vi "Data_get_joe_2.vi"() -> ()   [LabVIEW 2011]
uses:
  <vilib>/Utility/error.llb/DialogType.ctl
  <vilib>/Analysis/2dsp.llb/Real FFT.vi
  <vilib>/Analysis/NI_AALPro.lvlib
panel:
  in  "Automatic Overwrite?":bool
  out "f cur. (GHz)":i32
  in  "TDS VISA Port":refnum<visa-resource-name>="GPIB0::1::INSTR"
  in  "Chirp up to (GHz)":dbl
  in  "PauseB":bool caption="Pause"
  in  "Substr":bool
  out "tdsavges#":i32 caption="tds averaged:"
  in  "Auto":bool caption="Autosave"
  in  "FFT every#":u32=1 min=1 max=1000 step=1
  in  "#steps":u32=1 min=1 step=1
  in  "f step (MHz)":dbl=0.0003 min=0.00025 max=67.0 step=1e-06 format="%#.12f"
  in  "time/point":T1(ring)
  in  "time/div":T2(ring)
  out "Current sweep":u32=1 min=1 max=1000 step=1
  in  "Ext":string="ccd"
  in  "Name":string="trace"
  in  "Folder":path
  in  "#Sweeps":u32=1 min=1 max=1000 step=1
  in  "Ampl. (dBm)":dbl min=-135.0 max=30.0 step=0.5 format="%#_8g"
  in  "f start (GHz)":dbl=0.0003 min=0.00025 max=67.0 step=1e-06 format="%#.12f"
  in  "Start":bool
  in  "Quit":bool
  in  "Visa Port":refnum<visa-resource-name>="GPIB0::1::INSTR"
  out "read time (ms)":u32
  out "#points":u32
  out "Busy":bool
  in  "Chirp start (MHz)":ext=2.5
  in  "Filter up to (MHz)":ext=2.5
  in  "Amount of averagings":u32=10 min=1 step=1
  out "Data":dbl[](array[numeric])
  out "Frequency Domain Signal":cluster{ext[], dbl[]}(graph)
  out "FFT (Im)":dbl[](array[numeric])
  out "FFT (Re)":dbl[](array[numeric])
  out "Final array":ext[][](array[numeric])
  out "size(s)":i32
  out "Oscilloscope Data":dbl[](array[numeric])
  in  "Channel Number":u16=1
  out "Oscilloscope graph":dbl[](graph)
  in  "Stop":bool
  # "Oscilloscope TDS6124C"
  # "File Storage"
  # "PSG E8257D"
  # "Control"
  # "Spectrum data"
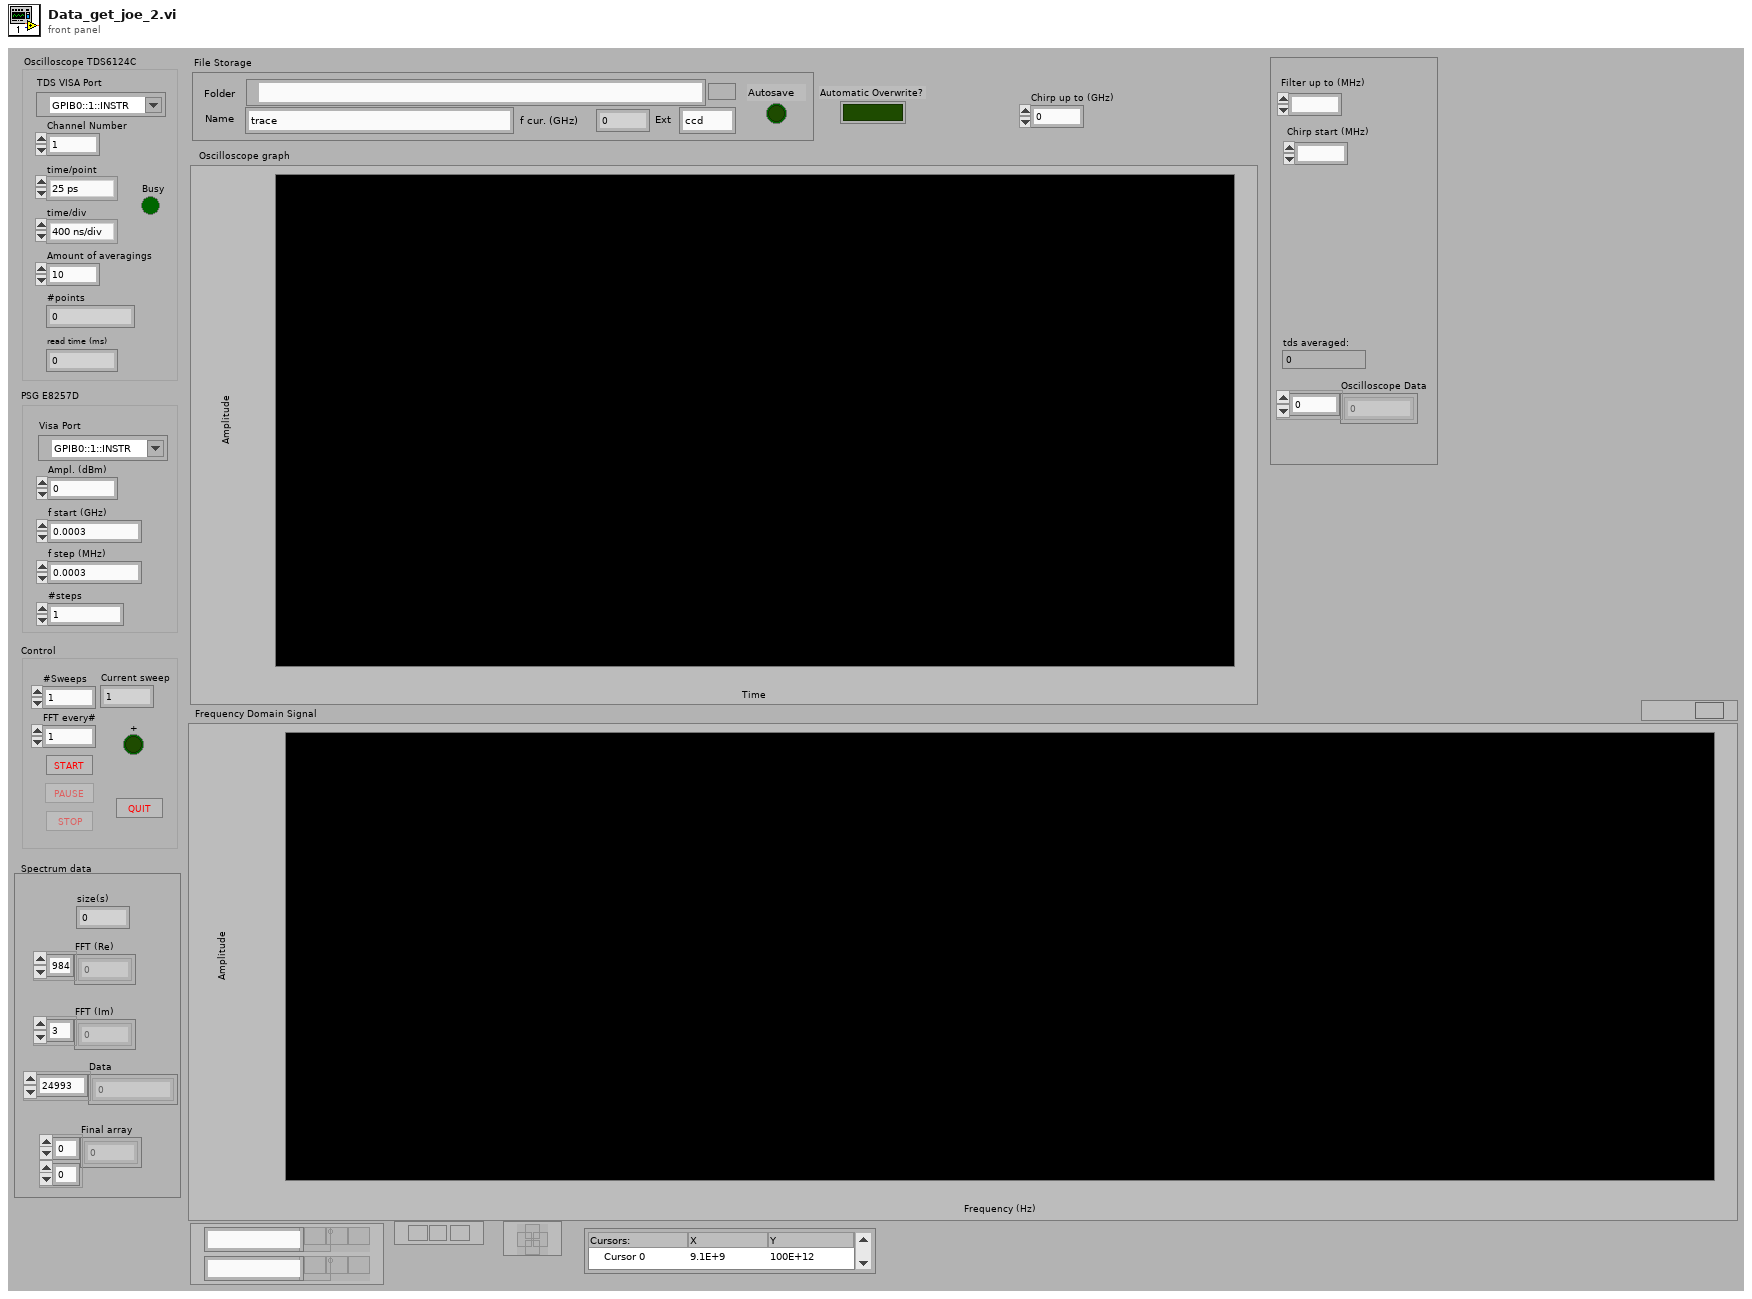
[diagram p1: front panel]
types:
  T1 = enum16{"25 ps", "50 ps", "100 ps", "200 ps", "400 ps", "800 ps", "2 ns"}
  T2 = enum16{"400 ns/div", "1 us/div", "2 us/div", "4 us/div", "10 us/div", "20 us/div"}
  T3 = enum8{"Enabled", "Disabled", "Disabled and Grayed Out"}
  T4 = enum16{"open", "replace", "create", "open or create", "replace or create", "replace or create with confirmation"}
  T5 = typedef "DialogType.ctl" = u16
  T6 = cluster{"Folder":path, "Name":string, "Ext":string}
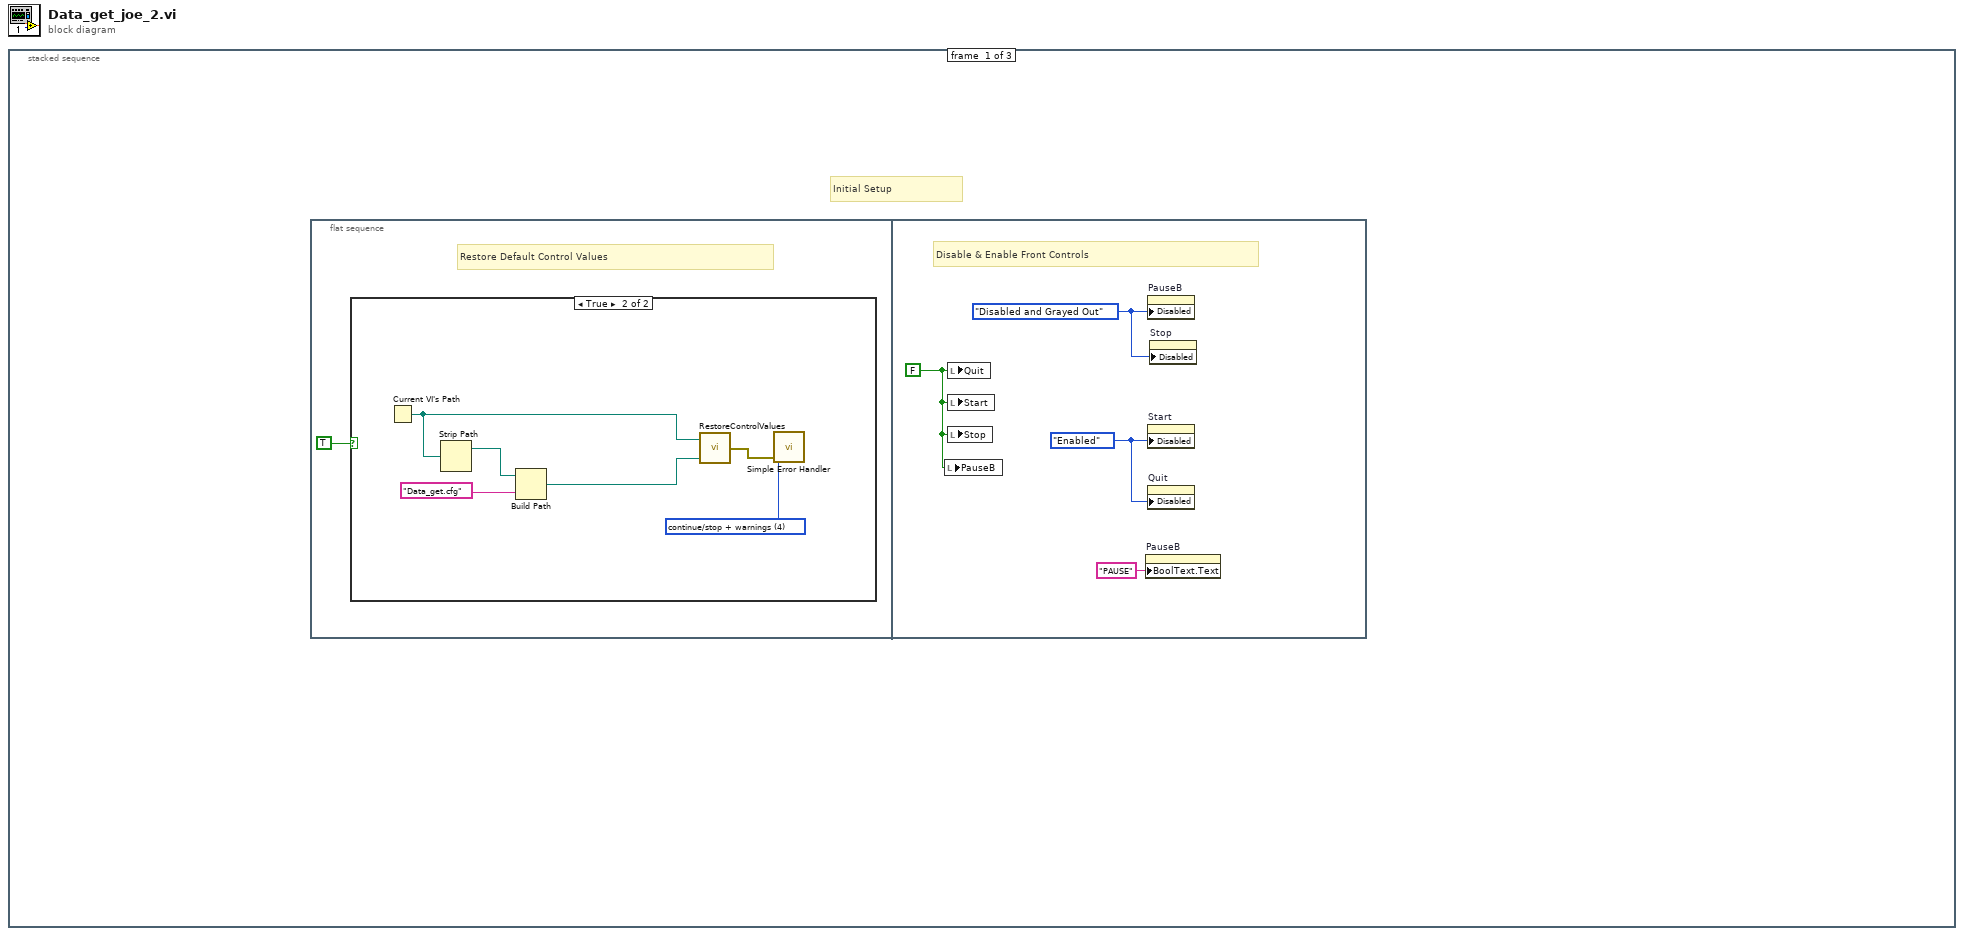
[diagram p0: block diagram]
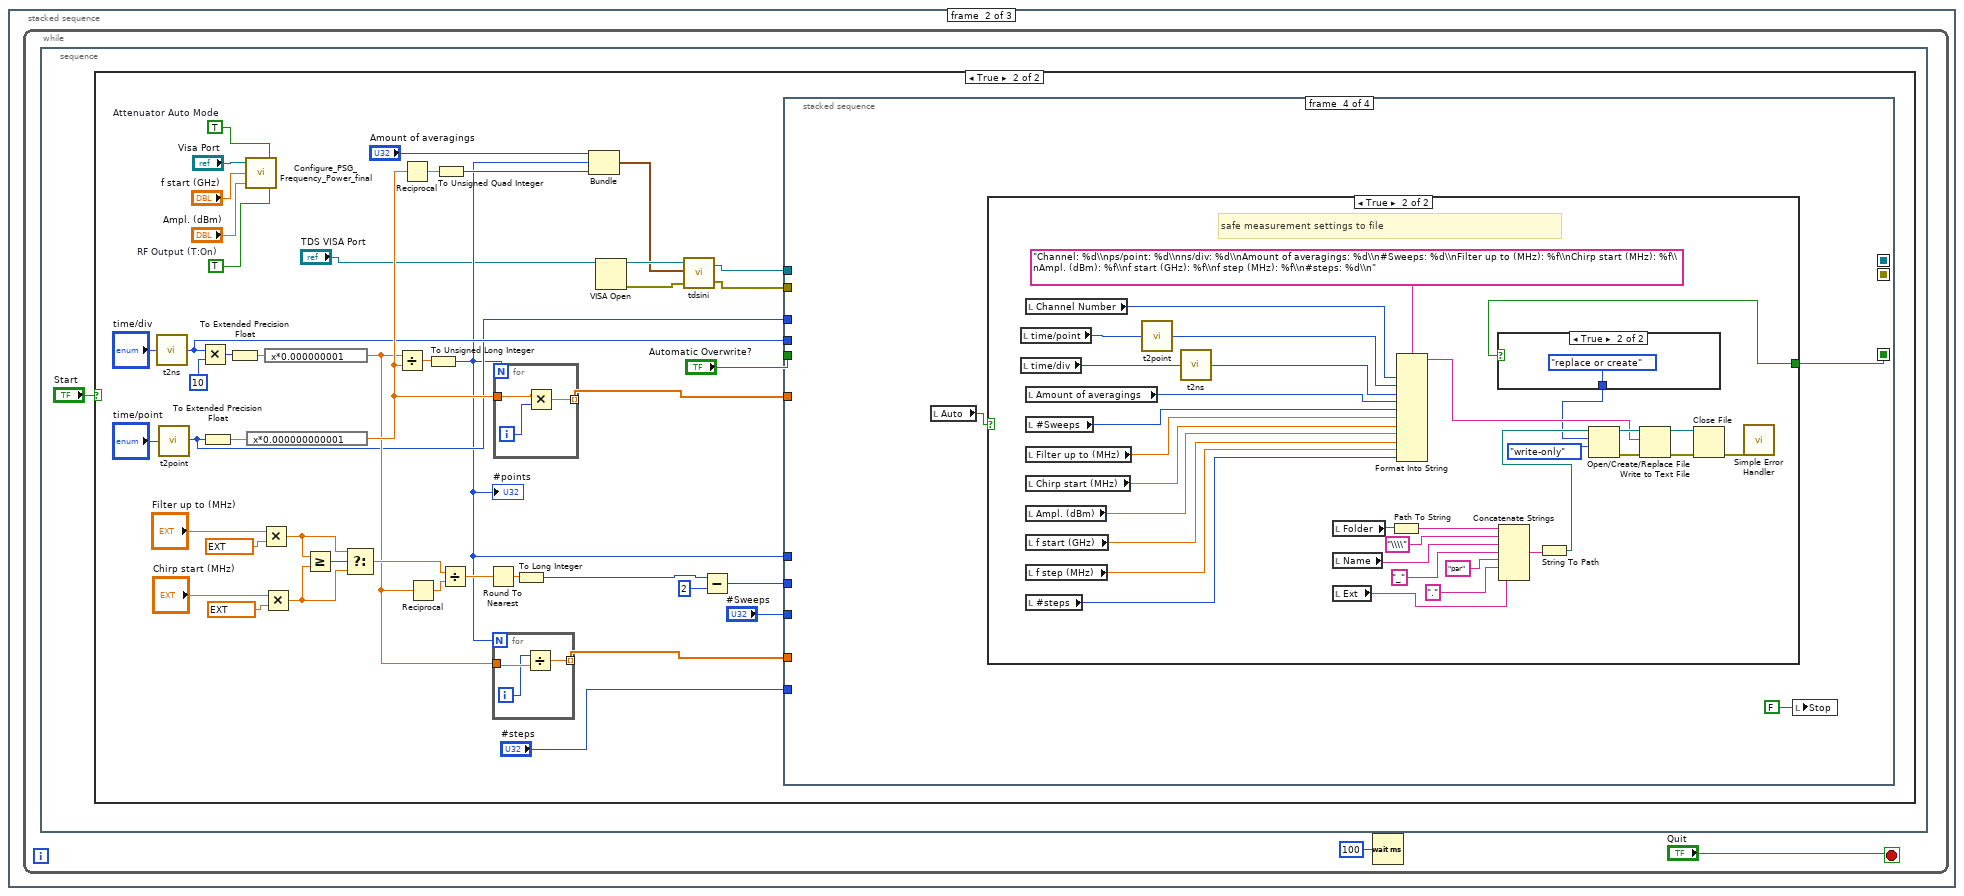
[diagram p3: hidden frame]
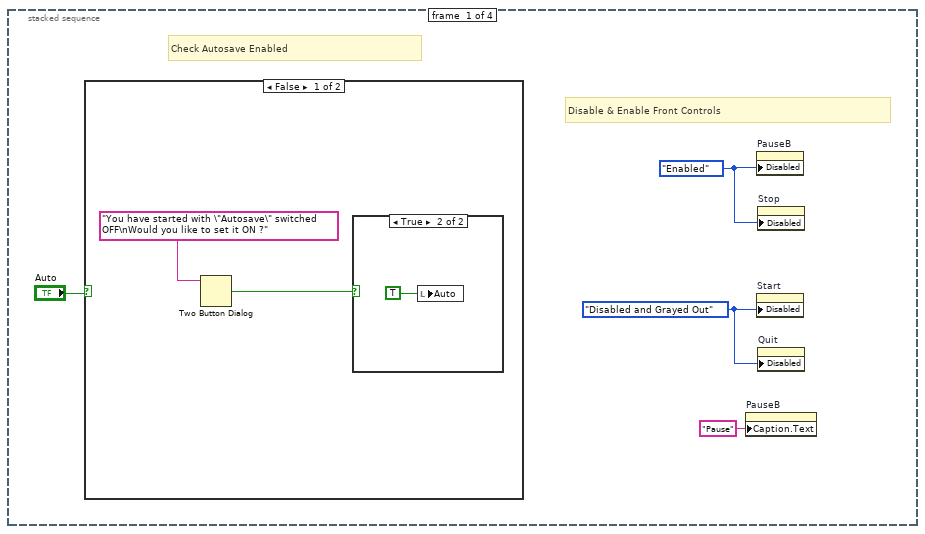
[diagram p5: hidden frame]
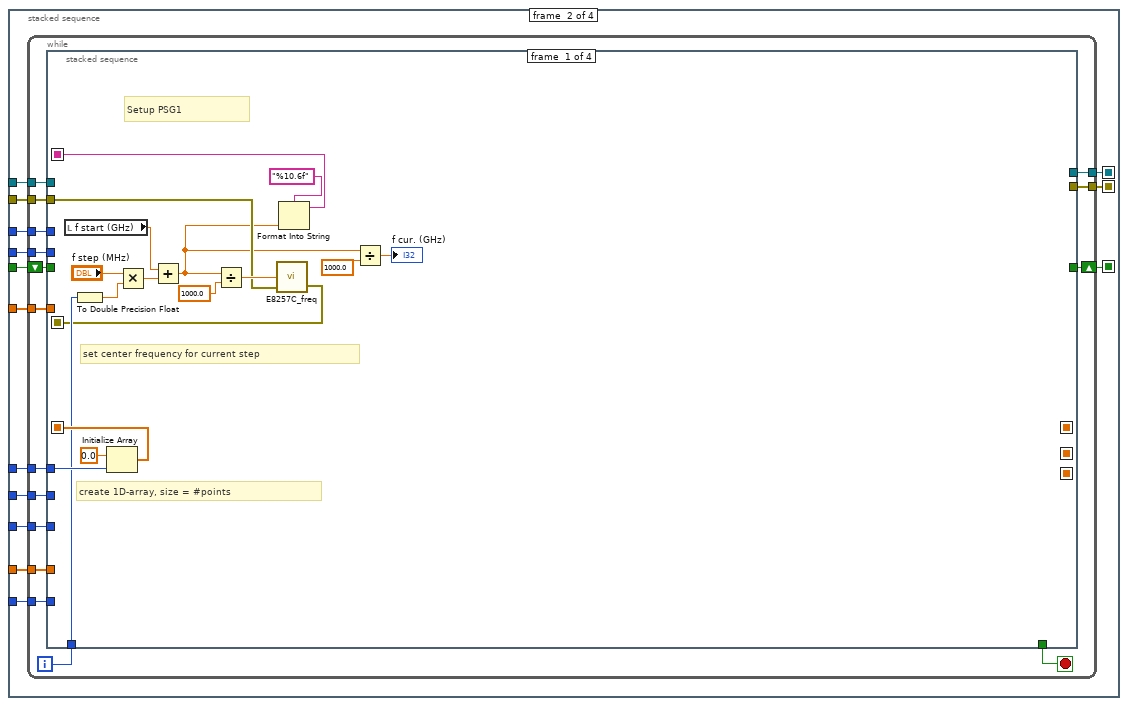
[diagram p8: hidden frame]
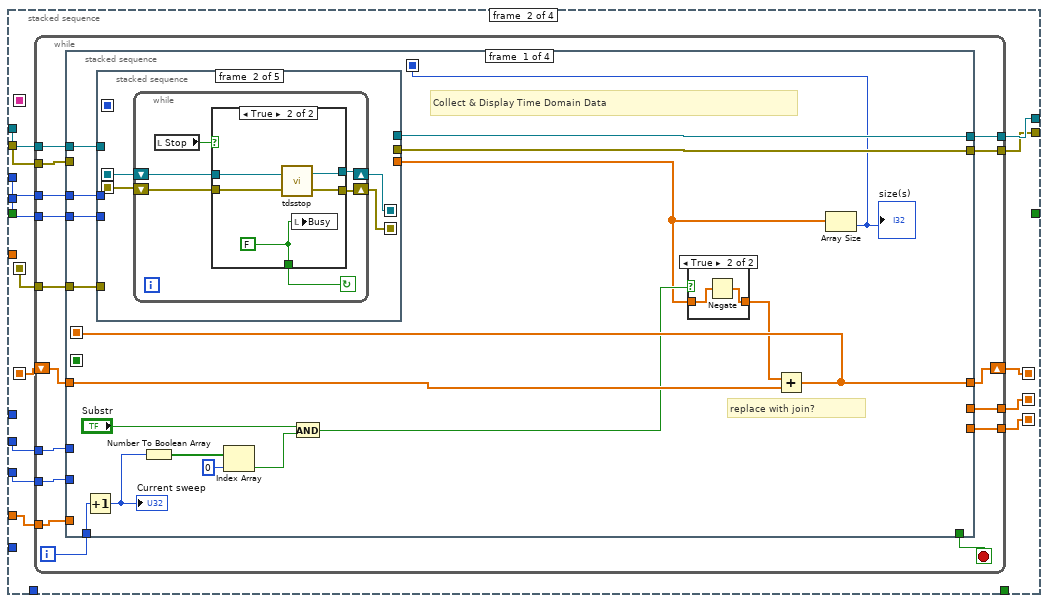
[diagram p9: hidden frame]
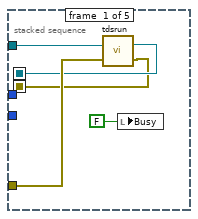
[diagram p11: hidden frame]
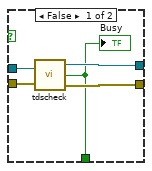
[diagram p12: hidden frame]
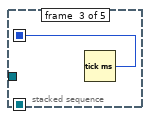
[diagram p13: hidden frame]
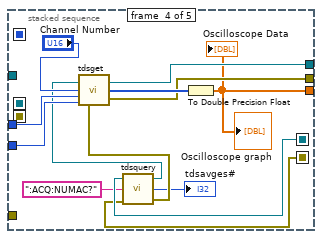
[diagram p14: hidden frame]
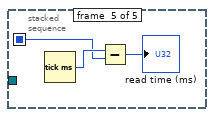
[diagram p15: hidden frame]
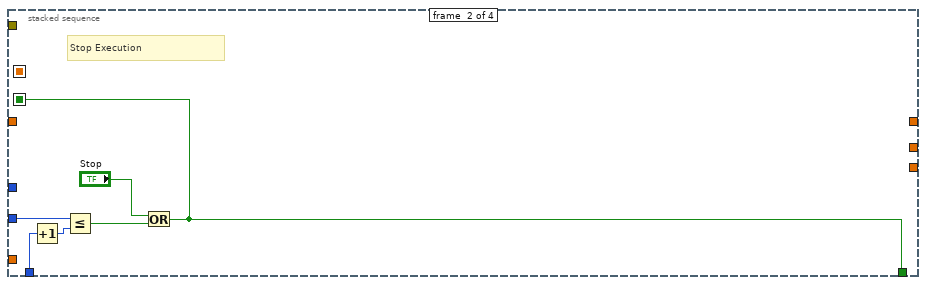
[diagram p16: hidden frame]
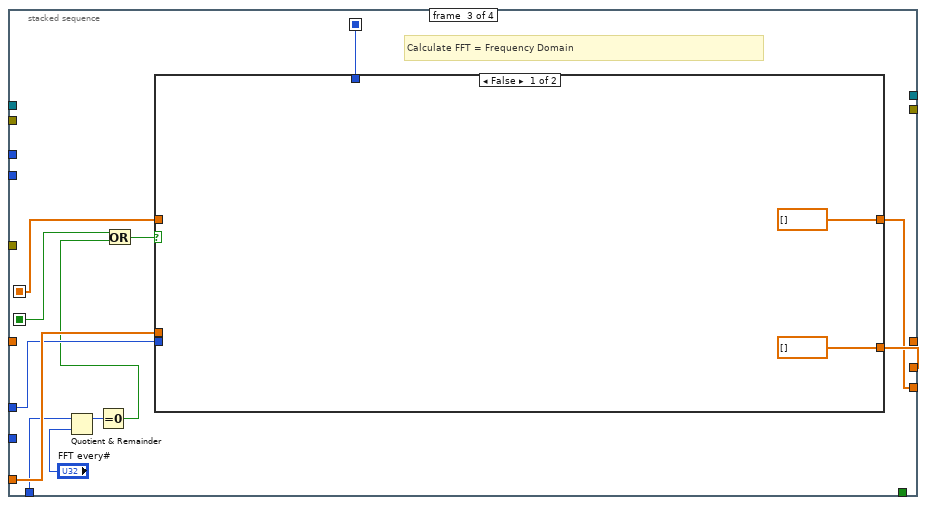
[diagram p17: hidden frame]
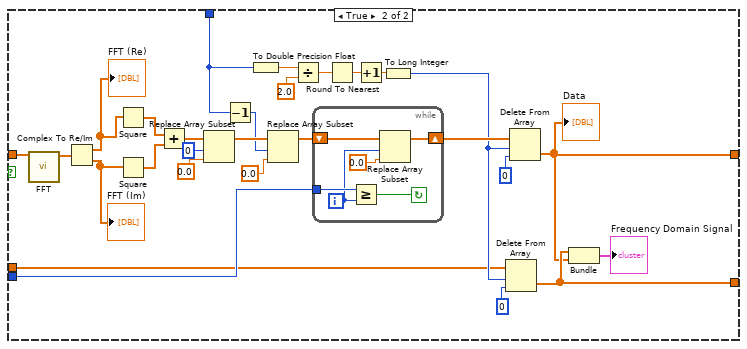
[diagram p18: hidden frame]
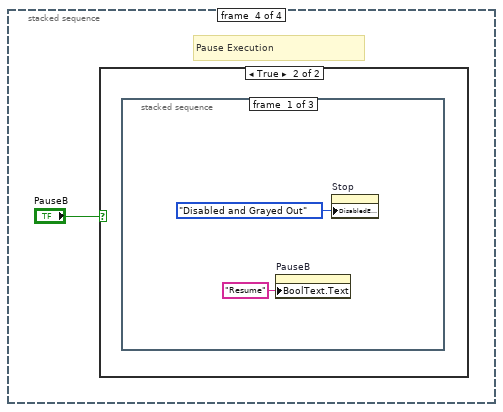
[diagram p19: hidden frame]
diagram:
  n1 = stacked-sequence {
    frame #0 {
      # "Initial Setup"
      n2 = flat-sequence {
        frame #0 {
          # "Restore Default Control Values"
          n3 = case shown="True" TRUE {
            frame False {
            }
            frame True {
              w2 = T5 4 items=["no dialog", "OK message", "continue or stop message", "OK message + warnings", "continue/stop + warnings"] ("type of dialog (OK msg:1)")
              n4 = Current VI's Path() -> (path=w3:path)
              n5 = Strip Path(path=w3) -> (stripped path=w4:path)  [unwired: 1 out]
              n6 = Build Path(base path=w4, name or relative path="Data_get.cfg") -> (appended path=w6:path)
              n7 = call "RestoreControlValues.vi"("file path"=w6, "vi path"=w3) -> ("error out"=w5:errorcluster)
              n8 = call <vilib>:"Simple Error Handler.vi"("type of dialog (OK msg:1)"=w2, "error in (no error)"=w5) -> ()  [unwired: 3 in, 5 out]
            }
          }
        }
        frame #1 {
          w10 = T3."Disabled and Grayed Out" ("Disabled")
          w8 = T3."Enabled" ("Disabled")
          w11 = FALSE ("Quit")
          # "Disable & Enable Front Controls"
          n9 = local write "PauseB"(w11) -> ()
          n10 = local write "Quit"(w11) -> ()
          n11 = local write "Start"(w11) -> ()
          n12 = local write "Stop"(w11) -> ()
          n13 = property on="PauseB" class="Bool (strict)"("BoolText.Text"="PAUSE" ("Boolean Text.Text")) -> ()  [unwired: 2 in, 2 out]
          n14 = property on="PauseB" class="Bool (strict)"("Disabled"=w10) -> ()  [unwired: 2 in, 2 out]
          n15 = property on="Start" class="Bool (strict)"("Disabled"=w8) -> ()  [unwired: 2 in, 2 out]
          n16 = property on="Quit" class="Bool (strict)"("Disabled"=w8) -> ()  [unwired: 2 in, 2 out]
          n17 = property on="Stop" class="Bool (strict)"("Disabled"=w10) -> ()  [unwired: 2 in, 2 out]
        }
      }
    }
    frame #1 {
      n18 = while {
        stop <- "Quit" stop-if-true
        n19 = stacked-sequence {
          frame #0 {
            n20 = case shown="True" "Start" {
              frame False {
              }
              frame True {
                w19 = TRUE  # Attenuator Auto Mode
                w16 = TRUE  # RF Output (T:On)
                n21 = call "t2ns.vi"("t/div"="time/div") -> ("ns/div"=w31:u32)
                n22 = call "t2point.vi"("t/point"="time/point") -> ("ps/point"=w29:u32)
                n23 = Multiply(x=w31, y=u32 10) -> (x*y=w54:u32)
                n24 = To Extended Precision Float(1:w29) -> (0:w51:ext)
                n25 = To Extended Precision Float(1:w54) -> (0:w52:ext)
                n26 = call "Configure_PSG_ Frequency_Power_final.vi"("RF Output (T:On)"=w16, "Attenuator Auto Mode (T:Enable)"=w19, "Power [dBm]"="Ampl. (dBm)", "Frequency [GHz]"="f start (GHz)", "VISA resource name"="Visa Port") -> ()
                n27 = expression code="x*0.000000000001"(w51) -> (w37:ext)
                n28 = Multiply(x="Filter up to (MHz)", y=ext 1000000.0) -> (x*y=w43:ext)
                n29 = Multiply(x="Chirp start (MHz)", y=ext 1000000.0) -> (x*y=w40:ext)
                n30 = expression code="x*0.000000001"(w52) -> (w33:ext)
                n31 = Greater Or Equal?(x=w43, y=w40) -> (x >= y?=w50:bool)
                n32 = Select(t=w43, s=w50, f=w40) -> (s? t:f=w48:ext)
                n33 = Divide(x=w33, y=w37) -> (x/y=w53:ext)
                n34 = Reciprocal(x=w37) -> (1/x=w35:ext)
                n35 = Reciprocal(x=w33) -> (1/x=w49:ext)
                n36 = To Unsigned Long Integer(number=w53) -> (unsigned 32bit integer=w27:u32)
                "#points" <- w27
                n37 = To Unsigned Quad Integer(1:w35) -> (0:w36:u64)
                n38 = Divide(x=w48, y=w49) -> (x/y=w47:ext)
                n39 = Round To Nearest(number=w47) -> (nearest integer value=w46:ext)
                n40 = for {
                  N: w27 -> [_]
                  tunnel: w33 -> [w459]
                  tunnel: [w460] -> w34 mode=indexing
                  i -> [w458]
                  n41 = Divide(x=w458, y=w459) -> (x/y=w460:ext)
                }
                n42 = for {
                  N: w27 -> [_]
                  tunnel: w37 -> [w463]
                  tunnel: [w462] -> w32 mode=indexing
                  i -> [w461]
                  n43 = Multiply(x=w463, y=w461) -> (x*y=w462:ext)
                }
                n44 = To Long Integer(number=w46) -> (32bit integer=w24:i32)
                n45 = Bundle("Amount of averagings"="Amount of averagings", w27, w36) -> (w38:cluster{"Amount of averagings ":u32, u32, u64})  [unwired: 1 in]
                n46 = VISA Open(VISA resource name="TDS VISA Port") -> (VISA resource name=w56:refnum<visa-resource-name>, error out=w57:errorcluster)  [unwired: 4 in]
                n47 = call "tdsini.vi"("Error In (No Error)"=w57, "Acq_par"=w38, "VISA Port In"=w56) -> ("Error Out"=w58:errorcluster, "VISA Port Out"=w59:refnum<visa-resource-name>)
                n48 = Subtract(x=w24, y=2) -> (x-y=w22:i32)
                n49 = stacked-sequence {
                  seq-local: [_ w73 _ _] -> [_ _ w419 _]
                  seq-local: [_ w72 _ _] -> [_ _ w418 _]
                  seq-local: [_ w67 _ _] -> [_ _ _ w420]
                  tunnel: w59 -> [_ w80 _ _]
                  tunnel: w58 -> [_ w79 _ _]
                  tunnel: w29 -> [_ w78 _ _]
                  tunnel: w31 -> [_ w77 _ _]
                  tunnel: w22 -> [_ w76 _ _]
                  tunnel: w34 -> [_ w75 _ _]
                  tunnel: "#Sweeps" -> [_ w74 _ _]
                  tunnel: w32 -> [_ w69 _ _]
                  tunnel: w27 -> [_ w71 _ _]
                  tunnel: "#steps" -> [_ w70 _ _]
                  tunnel: "Automatic Overwrite?" -> [_ w68 _ _]
                  frame #0 {
                    w61 = T3."Enabled" ("Disabled")
                    w60 = T3."Disabled and Grayed Out" ("Disabled")
                    # "Check Autosave Enabled"
                    # "Disable & Enable Front Controls"
                    n50 = case shown="False" "Auto" {
                      frame False {
                        n51 = Two Button Dialog(message="You have started with \"Autosave\" switched OFF\nWould you like to set it ON ?") -> (T button?=w64:bool)  [unwired: 2 in]
                        n52 = case shown="True" w64 {
                          frame False {
                          }
                          frame True {
                            n53 = local write "Auto"(TRUE) -> ()
                          }
                        }
                      }
                      frame True {
                      }
                    }
                    n54 = property on="PauseB" class="Bool (strict)"("Caption.Text"="Pause") -> ()  [unwired: 2 in, 2 out]
                    n55 = property on="PauseB" class="Bool (strict)"("Disabled"=w61) -> ()  [unwired: 2 in, 2 out]
                    n56 = property on="Start" class="Bool (strict)"("Disabled"=w60) -> ()  [unwired: 2 in, 2 out]
                    n57 = property on="Stop" class="Bool (strict)"("Disabled"=w61) -> ()  [unwired: 2 in, 2 out]
                    n58 = property on="Quit" class="Bool (strict)"("Disabled"=w60) -> ()  [unwired: 2 in, 2 out]
                  }
                  frame #1 {
                    n59 = while {
                      tunnel: w80 -> [w96]
                      tunnel: w79 -> [w95]
                      tunnel: w78 -> [w94]
                      tunnel: w77 -> [w93]
                      tunnel: w76 -> [w92]
                      tunnel: w75 -> [w91]
                      tunnel: w74 -> [w90]
                      tunnel: [w89] -> w73
                      tunnel: [w88] -> w72
                      tunnel: w71 -> [w87]
                      tunnel: w70 -> [w85]
                      tunnel: w69 -> [w83]
                      shift-right: [w81] -> w67
                      shift-left: w68 -> [w82]
                      i -> [w86]
                      stop <- w84 stop-if-true
                      n60 = stacked-sequence {
                        seq-local: [w112 _ _ _] -> [_ w118 _ _]
                        seq-local: [w102 _ _ _] -> [_ w117 _ _]
                        seq-local: [_ w116 _ _] -> [_ _ w274 _]
                        seq-local: [_ w115 _ _] -> [_ _ w273 _]
                        seq-local: [_ w114 _ _] -> [_ _ w272 _]
                        seq-local: [w100 _ _ _] -> [_ _ w271 _]
                        tunnel: w96 -> [_ w127 _ _]
                        tunnel: w95 -> [w103 w126 _ _]
                        tunnel: w94 -> [_ w125 _ _]
                        tunnel: w93 -> [_ w124 _ _]
                        tunnel: w92 -> [_ w123 _ _]
                        tunnel: w91 -> [_ w122 _ _]
                        tunnel: w90 -> [_ w121 _ _]
                        tunnel: [_ w120 _ _] -> w89
                        tunnel: [_ w119 _ _] -> w88
                        tunnel: w87 -> [w111 _ _ _]
                        tunnel: w86 -> [w106 _ _ w412]
                        tunnel: w85 -> [_ _ _ w411]
                        tunnel: [_ _ _ w410] -> w84
                        tunnel: w83 -> [_ _ w275 _]
                        tunnel: w82 -> [_ _ w269 _]
                        tunnel: [_ _ w268 _] -> w81
                        frame #0 {
                          # "Setup PSG1"
                          # "create 1D-array, size = #points"
                          # "set center frequency for current step"
                          n61 = local read "f start (GHz)"() -> (w104:dbl)
                          n62 = To Double Precision Float(number=w106) -> (double precision float=w107:dbl)
                          n63 = Initialize Array(0.0 ("element"), w111) -> (w112:dbl[])
                          n64 = Multiply(x="f step (MHz)", y=w107) -> (x*y=w105:dbl)
                          n65 = Add(x=w104, y=w105) -> (x+y=w98:dbl)
                          n66 = Divide(x=w98, y=1000.0) -> (x/y=w110:dbl)
                          n67 = call "E8257C_freq.vi"("error in"=w103, "Frequency GHz"=w110) -> ("error out"=w102:errorcluster)  [unwired: 1 in]
                          n68 = Format Into String(format string="%10.6f", w98) -> (resulting string=w100:string)  [unwired: 2 in, 1 out]
                          n69 = Divide(x=w98, y=1000.0) -> (x/y=→"f cur. (GHz)":dbl)
                        }
                        frame #1 {
                          n70 = while {
                            tunnel: [w140] -> w119
                            tunnel: [w141] -> w120
                            tunnel: w126 -> [w142]
                            tunnel: w127 -> [w143]
                            tunnel: w125 -> [w139]
                            tunnel: w124 -> [w138]
                            tunnel: w122 -> [w136]
                            tunnel: w123 -> [w137]
                            tunnel: w121 -> [w133]
                            shift-right: [w131] -> w116
                            shift-left: w118 -> [w132]
                            tunnel: [w130] -> w115
                            tunnel: w117 -> [w129]
                            tunnel: [w128] -> w114
                            i -> [w135]
                            stop <- w134 stop-if-true
                            n71 = stacked-sequence {
                              seq-local: [w153 _ _ _] -> [_ _ w224 _]
                              seq-local: [w154 _ _ _] -> [_ _ w223 _]
                              seq-local: [_ w207 _ _] -> [_ _ w214 _]
                              tunnel: w143 -> [w161 _ _ _]
                              tunnel: w142 -> [_ _ _ _]
                              tunnel: [w160 _ _ _] -> w141
                              tunnel: [w159 _ _ _] -> w140
                              tunnel: w139 -> [w158 _ _ _]
                              tunnel: w138 -> [w157 _ _ _]
                              tunnel: w137 -> [_ _ w221 _]
                              tunnel: w136 -> [_ _ w222 _]
                              tunnel: w135 -> [w152 w212 w218 _]
                              tunnel: [_ w207 _ _] -> w134
                              tunnel: w133 -> [_ w209 _ _]
                              tunnel: w132 -> [w156 _ _ _]
                              tunnel: [w154 _ _ _] -> w131
                              tunnel: [_ _ w220 _] -> w130
                              tunnel: w129 -> [w155 _ _ _]
                              tunnel: [_ _ w219 _] -> w128
                              frame #0 {
                                # "replace with join?"
                                # "Collect & Display Time Domain Data"
                                n72 = Increment(x=w152) -> (x+1=w144:i32)
                                "Current sweep" <- w144
                                n73 = stacked-sequence {
                                seq-local: [w167 _ _ _ _] -> [_ w173 _ _ _]
                                seq-local: [w166 _ _ _ _] -> [_ w172 _ _ _]
                                seq-local: [_ w170 _ _ _] -> [_ _ _ w195 _]
                                seq-local: [_ w171 _ _ _] -> [_ _ _ w196 _]
                                seq-local: [_ _ w190 _ _] -> [_ _ _ _ w205]
                                tunnel: w161 -> [w168 _ _ _ _]
                                tunnel: w155 -> [w169 _ _ _ _]
                                tunnel: [_ _ _ w202 _] -> w160
                                tunnel: [_ _ _ w201 _] -> w159
                                tunnel: w158 -> [_ _ _ w199 _]
                                tunnel: w157 -> [_ _ _ w198 _]
                                tunnel: [_ _ _ w197 _] -> w147
                                frame #0 {
                                n74 = call "tdsrun.vi"("Error In (No Error)"=w169, "VISA Port In"=w168) -> ("Error Out"=w166:errorcluster, "VISA Port Out"=w167:refnum<visa-resource-name>)
                                n75 = local write "Busy"(FALSE ("Busy")) -> ()
                                }
                                frame #1 {
                                n76 = while {
                                shift-right: [w177] -> w171
                                shift-left: w173 -> [w178]
                                shift-right: [w176] -> w170
                                shift-left: w172 -> [w179]
                                stop <- w175 continue-if-true
                                n77 = local read "Stop"() -> (w174:bool)
                                n78 = case shown="True" w174 {
                                tunnel: w179 -> [w184 w188]
                                tunnel: w178 -> [w183 w189]
                                tunnel: [w182 w186] -> w177
                                tunnel: [w181 w187] -> w176
                                tunnel: [w180 w185] -> w175
                                frame False {
                                n79 = call "tdscheck.vi"("VISA Port In"=w183, "Error In (No Error)"=w184) -> ("VISA Port Out"=w182:refnum<visa-resource-name>, "busy"=w180:bool, "Error Out"=w181:errorcluster)
                                "Busy" <- w180
                                }
                                frame True {
                                w185 = FALSE ("busy")
                                n80 = call "tdsstop.vi"("Error In (No Error)"=w188, "VISA Port In"=w189) -> ("Error Out"=w187:errorcluster, "VISA Port Out"=w186:refnum<visa-resource-name>)
                                n81 = local write "Busy"(w185) -> ()
                                }
                                }
                                }
                                }
                                frame #2 {
                                n82 = Tick Count (ms)() -> (millisecond timer value=w190:u32)
                                }
                                frame #3 {
                                n83 = call "tdsquery.vi"("Error In (No Error)"=w195, "String to TDS"=":ACQ:NUMAC?", "VISA Port In"=w196) -> ("Error Out"=w192:errorcluster, "number"=→"tdsavges#":i32, "VISA Port Out"=w193:refnum<visa-resource-name>)
                                n84 = call "tdsget.vi"("VISA Port In"=w193, "Channel Number"="Channel Number", "ps/point"=w199, "ns/div"=w198, "Error In (No Error)"=w192) -> ("VISA Port Out"=w202:refnum<visa-resource-name>, "TDS Data"=w203:u16[], "Error Out"=w201:errorcluster)  [unwired: 8 in]
                                n85 = To Double Precision Float(number=w203) -> (double precision float=w197:dbl[])
                                "Oscilloscope graph" <- w197
                                "Oscilloscope Data" <- w197
                                }
                                frame #4 {
                                n86 = Tick Count (ms)() -> (millisecond timer value=w206:u32)
                                n87 = Subtract(x=w206, y=w205) -> (x-y=→"read time (ms)":u32)
                                }
                                }
                                n88 = Number To Boolean Array(number=w144) -> (Boolean array=w151:bool[])
                                n89 = Index Array(array=w151, index=0) -> (element=w149:bool)
                                n90 = And(x="Substr", y=w149) -> (x .and. y?=w148:bool)
                                n91 = case shown="True" w148 {
                                tunnel: w147 -> [w162 w164]
                                tunnel: [w162 w163] -> w146
                                frame False {
                                }
                                frame True {
                                n92 = Negate(x=w164) -> (-x=w163:dbl[])
                                }
                                }
                                n93 = Add(x=w146, y=w156) -> (x+y=w154:dbl[])
                                n94 = Array Size(array=w147) -> (size(s)=w153:i32)
                                "size(s)" <- w153
                              }
                              frame #1 {
                                # "Stop Execution"
                                n95 = Increment(x=w212) -> (x+1=w208:i32)
                                n96 = Less Or Equal?(x=w209, y=w208) -> (x <= y?=w211:bool)
                                n97 = Or(x="Stop", y=w211) -> (x .or. y?=w207:bool)
                              }
                              frame #2 {
                                # "Calculate FFT = Frequency Domain"
                                n98 = Quotient & Remainder(x=w218, y="FFT every#") -> (x-y*floor(x/y)=w216:u32)  [unwired: 1 out]
                                n99 = Equal To 0?(x=w216) -> (x = 0?=w213:bool)
                                n100 = Or(x=w214, y=w213) -> (x .or. y?=w215:bool)
                                n101 = case shown="False" w215 {
                                tunnel: w224 -> [_ w232]
                                tunnel: w223 -> [_ w231]
                                tunnel: w222 -> [_ w227]
                                tunnel: w221 -> [_ w230]
                                tunnel: [ext[] [] w229] -> w220
                                tunnel: [dbl[] [] w228] -> w219
                                frame False {
                                }
                                frame True {
                                n102 = call-poly <vilib>:"FFT.vi"("X"=w231) -> ("FFT {X}"=w254:cdb[])  [unwired: 9 in, 1 out]
                                n103 = Complex To Re/Im(x + iy=w254) -> (x=w253:dbl[], y=w252:dbl[])
                                "FFT (Re)" <- w253
                                "FFT (Im)" <- w252
                                n104 = Square(x=w253) -> (x^2=w251:dbl[])
                                n105 = Square(x=w252) -> (x^2=w250:dbl[])
                                n106 = Add(x=w251, y=w250) -> (x+y=w246:dbl[])
                                n107 = Replace Array Subset(array=w246, new element=0.0 ("new element/subarray"), index=0) -> (w245:dbl[])
                                n108 = Decrement(x=w232) -> (x-1=w244:i32)
                                n109 = To Double Precision Float(number=w232) -> (double precision float=w240:dbl)
                                n110 = Replace Array Subset(array=w245, new element=0.0 ("new element/subarray"), index=w244) -> (w242:dbl[])
                                n111 = Divide(x=w240, y=2.0) -> (x/y=w238:dbl)
                                n112 = while {
                                tunnel: w230 -> [w259]
                                shift-right: [w257] -> w241
                                shift-left: w242 -> [w258]
                                i -> [w256]
                                stop <- w260 continue-if-true
                                n113 = Greater Or Equal?(x=w259, y=w256) -> (x >= y?=w260:bool)
                                n114 = Replace Array Subset(array=w258, new element=0.0 ("new element/subarray"), index=w256) -> (w257:dbl[])
                                }
                                n115 = Round To Nearest(number=w238) -> (nearest integer value=w237:dbl)
                                n116 = Increment(x=w237) -> (x+1=w236:dbl)
                                n117 = To Long Integer(number=w236) -> (32bit integer=w233:i32)
                                n118 = Delete From Array(array=w227, length=w233, index=0) -> (deleted portion=w229:ext[])  [unwired: 1 out]
                                n119 = Delete From Array(array=w241, length=w233, index=0) -> (deleted portion=w228:dbl[])  [unwired: 1 out]
                                "Data" <- w228
                                n120 = Bundle(w229, w228) -> (→"Frequency Domain Signal":cluster{ext[], dbl[]})  [unwired: 1 in]
                                }
                                }
                              }
                              frame #3 {
                                # "Pause Execution"
                                n121 = case shown="True" "PauseB" {
                                frame False {
                                }
                                frame True {
                                n122 = stacked-sequence {
                                frame #0 {
                                n123 = property on="PauseB" class="Bool (strict)"("BoolText.Text"="Resume" ("Caption.Text")) -> ()  [unwired: 2 in, 2 out]
                                n124 = property on="Stop" class="Bool (strict)"("DisabledEnum"=T3."Disabled and Grayed Out" ("Disabled")) -> ()  [unwired: 2 in, 2 out]
                                }
                                frame #1 {
                                n125 = while {
                                stop <- w265 continue-if-true
                                n126 = local read "PauseB"() -> (w265:bool)
                                n127 = Wait Until Next ms Multiple(millisecond multiple=u32 150) -> ()  [unwired: 1 out]
                                }
                                }
                                frame #2 {
                                n128 = property on="PauseB" class="Bool (strict)"("BoolText.Text"="Pause" ("Caption.Text")) -> ()  [unwired: 2 in, 2 out]
                                n129 = property on="Stop" class="Bool (strict)"("DisabledEnum"=T3."Enabled" ("Disabled")) -> ()  [unwired: 2 in, 2 out]
                                }
                                }
                                }
                                }
                              }
                            }
                          }
                        }
                        frame #2 {
                          # "Auto Safe?"
                          n130 = local read "Auto"() -> (w270:bool)
                          n131 = case shown="True" w270 {
                            tunnel: w275 -> [_ w283]
                            tunnel: w274 -> [_ w282]
                            tunnel: w273 -> [_ w281]
                            tunnel: w272 -> [_ w280]
                            tunnel: w271 -> [_ w279]
                            tunnel: w269 -> [_ w278]
                            tunnel: [FALSE w277] -> w268
                            frame False {
                            }
                            frame True {
                              n132 = stacked-sequence {
                                seq-local: [w284 _ _ _] -> [_ w308 _ _]
                                seq-local: [_ _ w362 _] -> [_ _ _ w402]
                                seq-local: [_ w294 _ _] -> [_ _ _ w393]
                                tunnel: w283 -> [_ w310 _ _]
                                tunnel: w282 -> [_ w297 _ _]
                                tunnel: w281 -> [_ _ _ w405]
                                tunnel: w280 -> [_ _ _ w404]
                                tunnel: w279 -> [w287 w296 w364 _]
                                tunnel: w278 -> [_ w300 _ _]
                                tunnel: [_ w294 _ _] -> w277
                                frame #0 {
                                # "create complete filename incl. path as a string"
                                n133 = Path To String(path="Folder") -> (string=w292:string)
                                n134 = Concatenate Strings(w292, "\\\\" ("string"), "Name", "_", "td", w287, ".", "Ext") -> (w284:string)
                                }
                                frame #1 {
                                # "(%e) = Scientific Notation"
                                n135 = Build Array(w310, w297) -> (w312:ext[][])
                                n136 = String To Path(string=w308) -> (path=w299:path)
                                n137 = case shown="False" w300 {
                                tunnel: w308 -> [w314 _]
                                tunnel: [w319 w360] -> w294
                                tunnel: [w317 T4."replace or create" ("operation (0:open)")] -> w302
                                tunnel: w300 -> [w318 w360]
                                tunnel: w299 -> [w316 w359]
                                tunnel: [w315 w359] -> w298
                                tunnel: w296 -> [w313 _]
                                frame False {
                                n138 = call "CheckFileExist.vi"("Path"=w314) -> ("File Exists"=w321:bool, "Overwrite File"=w320:bool)  [unwired: 1 in, 1 out]
                                n139 = case "check file existance" shown="True" w321 {
                                tunnel: w320 -> [_ w330]
                                tunnel: [w324 w328] -> w319
                                tunnel: w318 -> [w324 _]
                                tunnel: [T4."create" ("operation (0:open)") w329] -> w317
                                tunnel: w316 -> [w322 w327]
                                tunnel: [w322 w326] -> w315
                                tunnel: w313 -> [_ w325]
                                frame False {
                                # "file doesn't exist"
                                }
                                frame True {
                                # "file exists"
                                n140 = case shown="False" w330 {
                                tunnel: [w333 T4."replace or create" ("operation (0:open)")] -> w329
                                tunnel: [w334 TRUE] -> w328
                                tunnel: w327 -> [_ w356]
                                tunnel: [w331 w356] -> w326
                                tunnel: w325 -> [w332 _]
                                frame False {
                                # "file exists and should not be overwritten"
                                n141 = stacked-sequence {
                                tunnel: [_ _ FALSE] -> w334
                                tunnel: [_ _ T4."create" ("operation (0:open)")] -> w333
                                tunnel: w332 -> [_ w343 _]
                                tunnel: [_ w348 _] -> w331
                                frame #0 {
                                # "enter new file name"
                                n142 = local read "Folder"() -> (w342:path)
                                n143 = local read "Name"() -> (w341:string)
                                n144 = local read "Ext"() -> (w340:string)
                                n145 = Bundle("Folder"=w342, "Name"=w341, "Ext"=w340) -> (w339:T6)  [unwired: 1 in]
                                n146 = call "ChangeFileName.vi"("input par"=w339) -> ("output par"=w338:T6)  [unwired: 1 out]
                                n147 = Unbundle(w338) -> ("Folder"=w337:path, "Name"=w336:string, "Ext"=w335:string)
                                n148 = local write "Folder"(w337) -> ()
                                n149 = local write "Name"(w336) -> ()
                                n150 = local write "Ext"(w335) -> ()
                                }
                                frame #1 {
                                # "create new path"
                                n151 = local read "Ext"() -> (w345:string)
                                n152 = local read "Folder"() -> (w350:path)
                                n153 = local read "Name"() -> (w349:string)
                                n154 = Path To String(path=w350) -> (string=w353:string)
                                n155 = Concatenate Strings(w353, "\\\\" ("string"), w349, "_", "td", w343, ".", w345) -> (w344:string)
                                n156 = String To Path(string=w344) -> (path=w348:path)
                                }
                                frame #2 {
                                }
                                }
                                }
                                frame True {
                                # "overwrite existing file"
                                }
                                }
                                }
                                }
                                }
                                frame True {
                                }
                                }
                                n157 = Transpose 2D Array(2D array=w312) -> (transposed array=w309:ext[][])
                                n158 = Array To Spreadsheet String(array=w309, 3:"%e") -> (spreadsheet string=w301:string)  [unwired: 1 in]
                                n159 = Open/Create/Replace File(file path (use dialog)=w298, operation (0:open)=w302, access (0:read/write)=enum16{"read/write", "read-only", "write-only"}."write-only") -> (refnum out=w304:refnum<file>, error out=w307:errorcluster)  [unwired: 3 in, 1 out]
                                n160 = Write to Text File(file (use dialog)=w304, text=w301, error in=w307) -> (refnum out=w305:refnum<file>, error out=w306:errorcluster)  [unwired: 1 in, 1 out]
                                n161 = Close File(refnum=w305, error in=w306) -> (error out=w295:errorcluster)  [unwired: 1 out]
                                n162 = call <vilib>:"Simple Error Handler.vi"("error in (no error)"=w295) -> ()  [unwired: 4 in, 5 out]
                                }
                                frame #2 {
                                n163 = local read "Folder"() -> (w366:path)
                                n164 = local read "Name"() -> (w365:string)
                                n165 = local read "Ext"() -> (w363:string)
                                n166 = Path To String(path=w366) -> (string=w372:string)
                                n167 = Concatenate Strings(w372, "\\\\" ("string"), w365, "_") -> (w367:string)
                                n168 = Concatenate Strings(w367, "sd", w364, ".", w363) -> (w362:string)
                                }
                                frame #3 {
                                n169 = Multiply(x="Chirp up to (GHz)", y=1000000000.0) -> (x*y=w374:dbl)
                                n170 = To Extended Precision Float(1:w374) -> (0:w373:ext)
                                n171 = To Extended Precision Float(1:w404) -> (0:w406:ext[])
                                n172 = Build Array(w405, w406) -> (w403:ext[][])
                                n173 = String To Path(string=w402) -> (path=w395:path)
                                n174 = case shown="True" w393 {
                                tunnel: [T4."replace or create with confirmation" ("operation (0:open)") T4."replace or create" ("operation (0:open)")] -> w394
                                frame False {
                                }
                                frame True {
                                }
                                }
                                n175 = Transpose 2D Array(2D array=w403) -> (transposed array=w376:ext[][])
                                n176 = Index Array(array=w376, index (col)=0 ("disabled index (col)")) -> (element=w386:ext[])  [unwired: 1 in]
                                n177 = Index Array(array=w386, index=1) -> (element=w388:ext)
                                n178 = Index Array(array=w386, index=0) -> (element=w387:ext)
                                n179 = Subtract(x=w388, y=w387) -> (x-y=w383:ext)
                                n180 = Divide(x=w373, y=w383) -> (x/y=w380:ext)
                                n181 = Round To Nearest(number=w380) -> (nearest integer value=w382:ext)
                                n182 = To Long Integer(number=w382) -> (32bit integer=w381:i32)
                                n183 = Increment(x=w381) -> (x+1=w377:i32)
                                n184 = Array Subset(array=w376, index (row)=0 ("index"), length (row)=w377, index (col)=0 ("index"), length (col)=w377) -> (w375:ext[][])
                                "Final array" <- w375
                                n185 = Array To Spreadsheet String(array=w375, 3:"%e") -> (spreadsheet string=w396:string)  [unwired: 1 in]
                                n186 = Open/Create/Replace File(file path (use dialog)=w395, operation (0:open)=w394, access (0:read/write)=enum16{"read/write", "read-only", "write-only"}."write-only") -> (refnum out=w398:refnum<file>, error out=w401:errorcluster)  [unwired: 3 in, 1 out]
                                n187 = Write to Text File(file (use dialog)=w398, text=w396, error in=w401) -> (refnum out=w399:refnum<file>, error out=w400:errorcluster)  [unwired: 1 in, 1 out]
                                n188 = Close File(refnum=w399, error in=w400) -> (error out=w392:errorcluster)  [unwired: 1 out]
                                n189 = call <vilib>:"Simple Error Handler.vi"("error in (no error)"=w392) -> ()  [unwired: 4 in, 5 out]
                                }
                              }
                            }
                          }
                        }
                        frame #3 {
                          n190 = Increment(x=w412) -> (x+1=w414:i32)
                          n191 = Less Or Equal?(x=w411, y=w414) -> (x <= y?=w415:bool)
                          n192 = local read "Stop"() -> (w413:bool)
                          n193 = Or(x=w413, y=w415) -> (x .or. y?=w410:bool)
                        }
                      }
                    }
                  }
                  frame #2 {
                    w417 = T3."Disabled and Grayed Out" ("Disabled")
                    w416 = T3."Enabled" ("Disabled")
                    n194 = property on="Quit" class="Bool (strict)"("Disabled"=w416) -> ()  [unwired: 2 in, 2 out]
                    n195 = property on="PauseB" class="Bool (strict)"("Disabled"=w417) -> ()  [unwired: 2 in, 2 out]
                    n196 = property on="Stop" class="Bool (strict)"("Disabled"=w417) -> ()  [unwired: 2 in, 2 out]
                    n197 = property on="Start" class="Bool (strict)"("Disabled"=w416) -> ()  [unwired: 2 in, 2 out]
                    n198 = VISA Close(VISA resource name=w419, error in (no error)=w418) -> ()  [unwired: 1 out]
                  }
                  frame #3 {
                    n199 = local read "Auto"() -> (w421:bool)
                    n200 = case shown="True" w421 {
                      tunnel: w420 -> [_ w424]
                      frame False {
                      }
                      frame True {
                        # "safe measurement settings to file"
                        n201 = local read "time/point"() -> (w453:T1)
                        n202 = local read "time/div"() -> (w452:T2)
                        n203 = local read "Channel Number"() -> (w454:u16)
                        n204 = local read "Amount of averagings"() -> (w451:u32)
                        n205 = local read "#Sweeps"() -> (w450:u32)
                        n206 = local read "Filter up to (MHz)"() -> (w449:ext)
                        n207 = local read "Chirp start (MHz)"() -> (w448:ext)
                        n208 = local read "Ampl. (dBm)"() -> (w447:dbl)
                        n209 = local read "f start (GHz)"() -> (w444:dbl)
                        n210 = local read "f step (MHz)"() -> (w443:dbl)
                        n211 = local read "#steps"() -> (w442:u32)
                        n212 = call "t2point.vi"("t/point"=w453) -> ("ps/point"=w445:u32)
                        n213 = call "t2ns.vi"("t/div"=w452) -> ("ns/div"=w446:u32)
                        n214 = local read "Folder"() -> (w438:path)
                        n215 = local read "Name"() -> (w437:string)
                        n216 = local read "Ext"() -> (w434:string)
                        n217 = Path To String(path=w438) -> (string=w441:string)
                        n218 = Format Into String(format string="Channel: %d\\nps/point: %d\\nns/div: %d\\nAmount of averagings: %d\\n#Sweeps: %d\\nFilter up to (MHz): %f\\nChirp start (MHz): %f\\nAmpl. (dBm): %f\\nf start (GHz): %f\\nf step (MHz): %f\\n#steps: %d\\n", w454, w445, w446, w451, w450, w449, w448, w447, w444, w443, w442) -> (resulting string=w425:string)  [unwired: 2 in, 1 out]
                        n219 = case shown="True" w424 {
                          tunnel: [T4."replace or create with confirmation" ("operation (0:open)") T4."replace or create" ("operation (0:open)")] -> w423
                          frame False {
                          }
                          frame True {
                          }
                        }
                        n220 = Concatenate Strings(w441, "\\\\" ("string"), w437, "_", "par", ".", w434) -> (w433:string)
                        n221 = String To Path(string=w433) -> (path=w427:path)
                        n222 = Open/Create/Replace File(file path (use dialog)=w427, operation (0:open)=w423, access (0:read/write)=enum16{"read/write", "read-only", "write-only"}."write-only") -> (refnum out=w429:refnum<file>, error out=w432:errorcluster)  [unwired: 3 in, 1 out]
                        n223 = Write to Text File(file (use dialog)=w429, text=w425, error in=w432) -> (refnum out=w430:refnum<file>, error out=w431:errorcluster)  [unwired: 1 in, 1 out]
                        n224 = Close File(refnum=w430, error in=w431) -> (error out=w428:errorcluster)  [unwired: 1 out]
                        n225 = call <vilib>:"Simple Error Handler.vi"("error in (no error)"=w428) -> ()  [unwired: 4 in, 5 out]
                      }
                    }
                    n226 = local write "Stop"(FALSE ("Stop")) -> ()
                  }
                }
              }
            }
          }
        }
        n227 = Wait (ms)(milliseconds to wait=u32 100) -> ()  [unwired: 1 out]
      }
    }
    frame #2 {
      n228 = Current VI's Path() -> (path=w464:path)
      n229 = Strip Path(path=w464) -> (stripped path=w465:path)  [unwired: 1 out]
      n230 = Build Path(base path=w465, name or relative path="Data_get.cfg") -> (appended path=w467:path)
      n231 = call "SaveControlValues.vi"("file path"=w467, "vi path"=w464) -> ("error out"=w466:errorcluster)
      n232 = call <vilib>:"Simple Error Handler.vi"("error in (no error)"=w466) -> ()  [unwired: 4 in, 5 out]
    }
  }
